vi "Array-Decimate.vi"(9 "Decimation Step":i32, 11 "Array":dbl[](array[numeric])) -> (3 "Decimated Array":dbl[](array[numeric]))   [LabVIEW 2020]
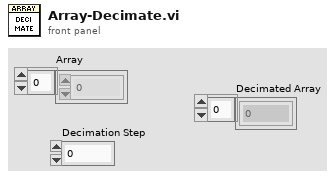
[diagram p1: front panel]
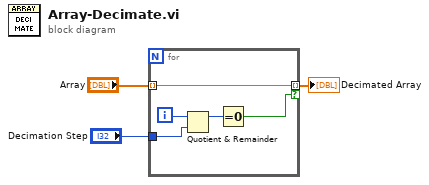
[diagram p0: block diagram]
diagram:
  n1 = for {
    tunnel: "Array" -> [w5] mode=indexing
    tunnel: "Decimation Step" -> [w7]
    tunnel: [w5] -> w1 mode=indexing if=w4
    i -> [w8]
    n2 = Quotient & Remainder(x=w8, y=w7) -> (x-y*floor(x/y)=w6:i32)  [unwired: 1 out]
    n3 = Equal To 0?(x=w6) -> (x = 0?=w4:bool)
  }
  "Decimated Array" <- w1
